vi "Stem-and-Leaf - Format.vi"(10 "Number of digits to fill the display":i32=64, 11 "String In":string="\r\n") -> (3 "String Formatted":string)   [LabVIEW 2023]
doc: "Parses the incoming string so that the | character properly lines up as a vertical line. This VI also truncates rows with long strings that might wrap the string indicator displaying the output to preserve the strict alignment of the display."
panel:
  # "This truncates the string and prevents the wrapping of text at the edge of the string."
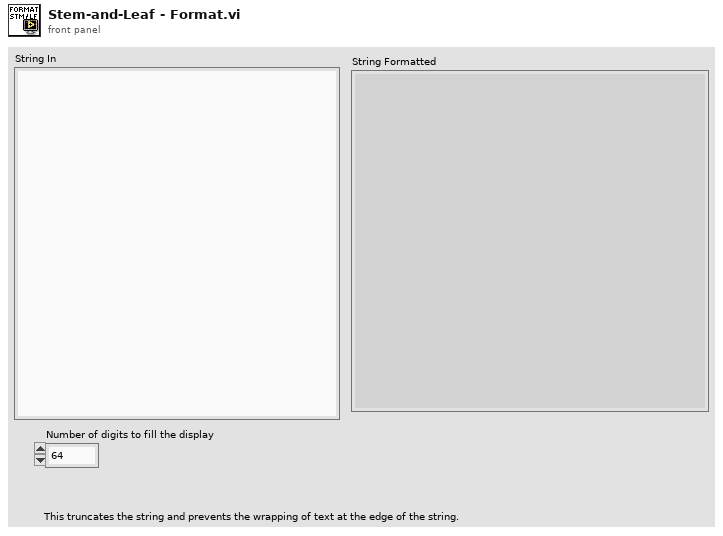
[diagram p1: front panel]
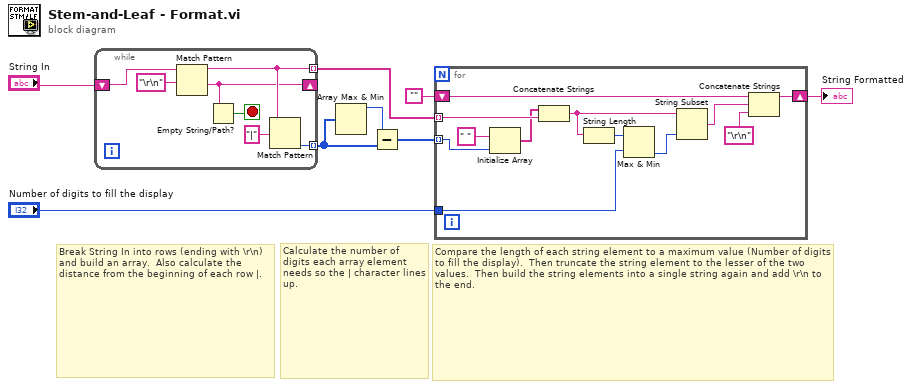
[diagram p0: block diagram]
diagram:
  # "Compare the length of each string element to a maximum value (Number of digits to fill the display).  Then truncate the string element to the lesser of the two values.  Then build the string elements into a single string again and add \\r\\n to the end."
  # "Calculate the number of digits each array element needs so the | character lines up."
  # "Break String In into rows (ending with \\r\\n) and build an array.  Also calculate the distance from the beginning of each row |."
  n1 = while {
    shift-right: [w9] -> _
    shift-left: "String In" -> [w13]
    tunnel: [w11] -> w4 mode=indexing
    tunnel: [w10] -> w6 mode=indexing
    stop <- w15 stop-if-true
    n2 = Match Pattern(string=w13, regular expression="\r\n" ("search string")) -> (before substring=w11:string, after substring=w9:string)  [unwired: 1 in, 2 out]
    n3 = Empty String/Path?(string/path=w9) -> (empty?=w15:bool)
    n4 = Match Pattern(string=w11, regular expression="|" ("search string")) -> (offset past match=w10:i32)  [unwired: 1 in, 3 out]
  }
  n5 = Array Max & Min(array=w6) -> (max value=w7:i32)  [unwired: 3 out]
  n6 = Subtract(x=w7, y=w6) -> (x-y=w5:i32[])
  n7 = for {
    tunnel: w5 -> [w18] mode=indexing
    tunnel: w4 -> [w27] mode=indexing
    shift-right: [w23] -> w3
    shift-left: "" -> [w22]
    tunnel: "Number of digits to fill the display" -> [w19]
    n8 = Initialize Array(" " ("string"), w18) -> (w16:string[])
    n9 = Concatenate Strings(w16, w27) -> (w25:string)
    n10 = String Length(string=w25) -> (length=w26:i32)
    n11 = Max & Min(x=w26, y=w19) -> (min(x,y)=w24:i32)  [unwired: 1 out]
    n12 = String Subset(string=w25, length (rest)=w24) -> (substring=w20:string)  [unwired: 1 in]
    n13 = Concatenate Strings(w22, w20, "\r\n" ("search string")) -> (w23:string)
  }
  "String Formatted" <- w3
